vi "Roop_Polymer_string_to_timestamp.vi"(10 "error in (no error)":errorcluster, 11 "String":string) -> (2 "error out":errorcluster, 3 "Time Stamp":timestamp format="%<%.3X\n%Y/%m/%d>T", 5 "time":string)   [LabVIEW 2017]
uses:
  <vilib>/Utility/miscctls.llb/LVDateTimeRec.ctl
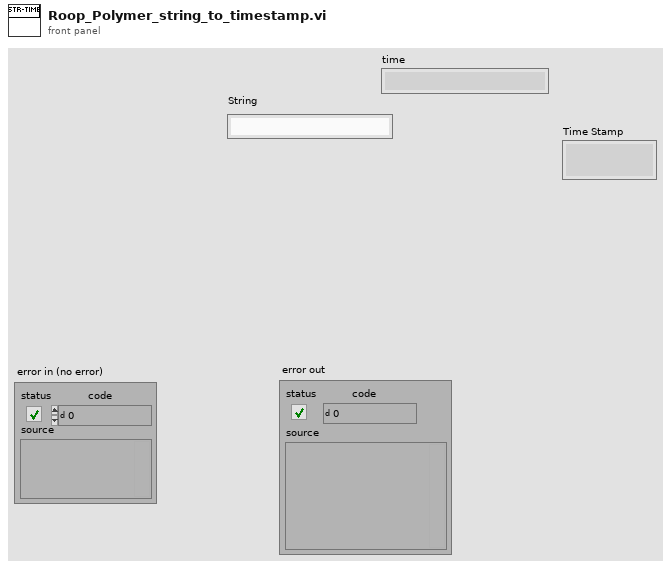
[diagram p1: front panel]
types:
  T1 = typedef "LVDateTimeRec.ctl" = cluster{"fractional second":dbl, "second":i32, "minute":i32, "hour":i32, "day of month":i32, "month":i32, "year":i32, "day of week":i32, "day of year":i32, "DST":i32}
  T2 = cluster{"second":i32, "minute":i32, "hour":i32, "day of month":i32, "month":i32, "year":i32, "day of week":i32, "day of year":i32, "is DST":i32}
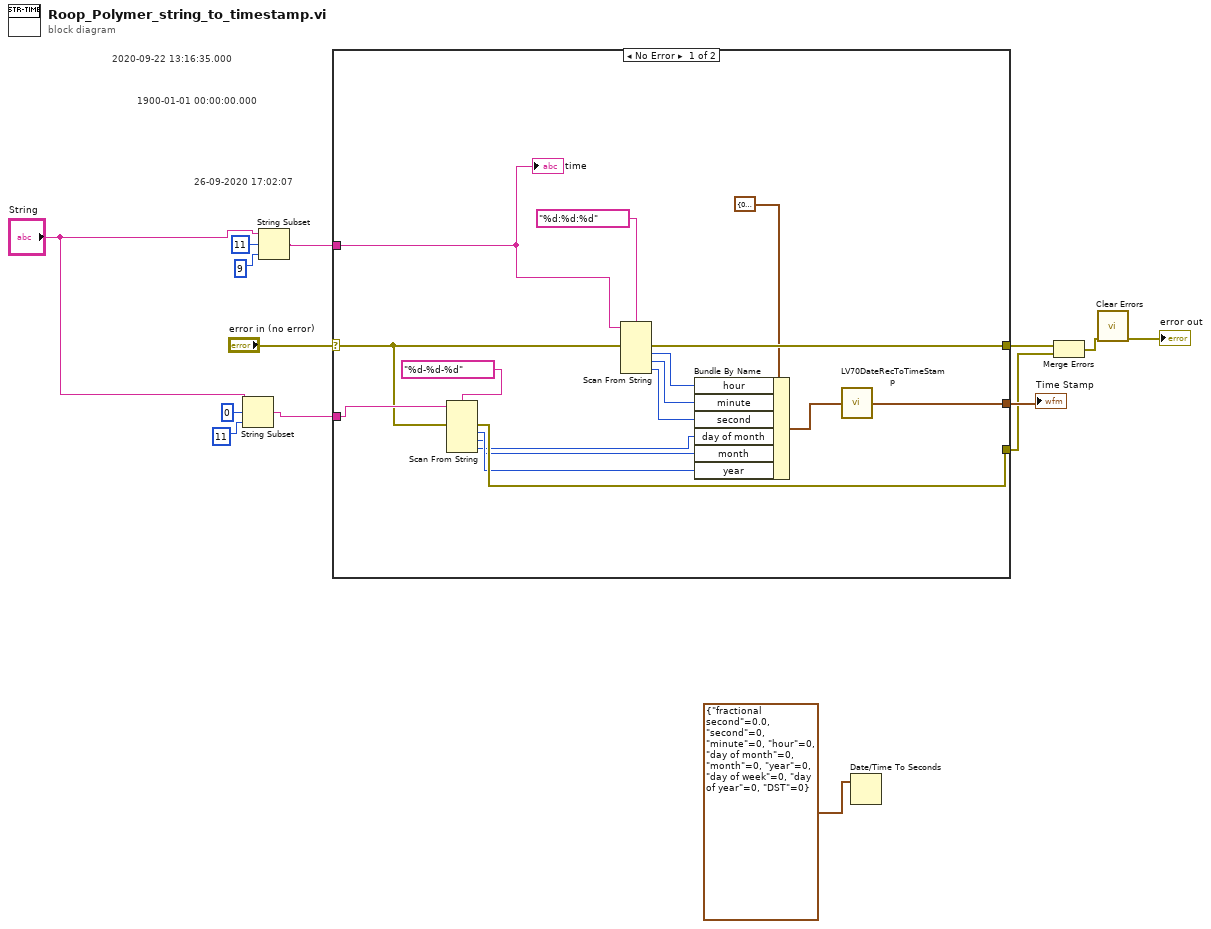
[diagram p0: block diagram]
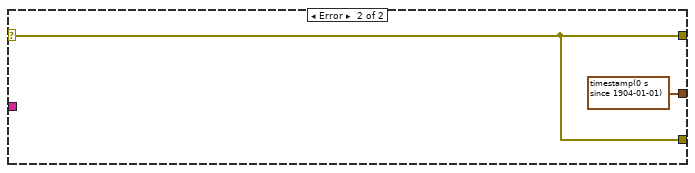
[diagram p2: hidden frame]
diagram:
  # "26-09-2020 17:02:07"
  # "2020-09-22 13:16:35.000"
  # "1900-01-01 00:00:00.000"
  n1 = String Subset(string="String", offset (0)=0, length (rest)=11 ("length (rest)")) -> (substring=w5:string)
  n2 = String Subset(string="String", offset (0)=11, length (rest)=9 ("length (rest)")) -> (substring=w8:string)
  n3 = case shown="No Error" "error in (no error)" {
    selector: "error in (no error)" -> [w19 w31]
    tunnel: [w30 w31] -> w13
    tunnel: w8 -> [w22 _]
    tunnel: [w24 timestamp(0 s since 1904-01-01) ("Time Stamp")] -> w12
    tunnel: w5 -> [w20 _]
    tunnel: [w18 w31] -> w2
    frame No Error {
      n4 = Scan From String(format string="%d-%d-%d", input string=w20, error in=w19) -> (error out=w18:errorcluster, output 1=w17:i32, output 2=w16:i32, output 3=w15:i32)  [unwired: 4 in, 2 out]
      n5 = Scan From String(format string="%d:%d:%d", input string=w22, error in=w19) -> (error out=w30:errorcluster, output 1=w27:i32, output 2=w26:i32, output 3=w25:i32)  [unwired: 4 in, 2 out]
      n6 = Bundle By Name(cluster=T2 {"second"=0, "minute"=0, "hour"=0, "day of month"=1, "month"=1, "year"=2018, "day of week"=0, "day of year"=0, "is DST"=0} ("date time rec"), "hour"=w27, "minute"=w26, "second"=w25, "day of month"=w15, "month"=w16, "year"=w17) -> (w23:T2)
      n7 = call <vilib>:"LV70DateRecToTimeStamp.vi"("date time rec"=w23) -> ("Time Stamp"=w24:timestamp)
      "time" <- w22
    }
    frame Error {
    }
  }
  "Time Stamp" <- w12
  n8 = Date/Time To Seconds(2:T1 {"fractional second"=0.0, "second"=0, "minute"=0, "hour"=0, "day of month"=0, "month"=0, "year"=0, "day of week"=0, "day of year"=0, "DST"=0} ("date time rec")) -> ()  [unwired: 1 in, 1 out]
  n9 = Merge Errors(w13, w2) -> (w3:errorcluster)
  n10 = call <vilib>:"Clear Errors.vi"("error in (no error)"=w3) -> ("error out"=→"error out":errorcluster)  [unwired: 5 in, 1 out]
